vi "SetUpPlotLegend_V0.vi"(1 "Comment":string[](array[string]), 2 "Index":i32[](array[numeric]), 3 "Graph":refnum<vi>) -> ()   [LabVIEW 2021]
panel:
  in  "Graph 2":refnum<vi>
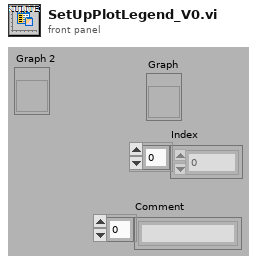
[diagram p1: front panel]
types:
  T1 = cluster{"Start":dbl, "Delta x":dbl, "Data Array out":sgl[][]}
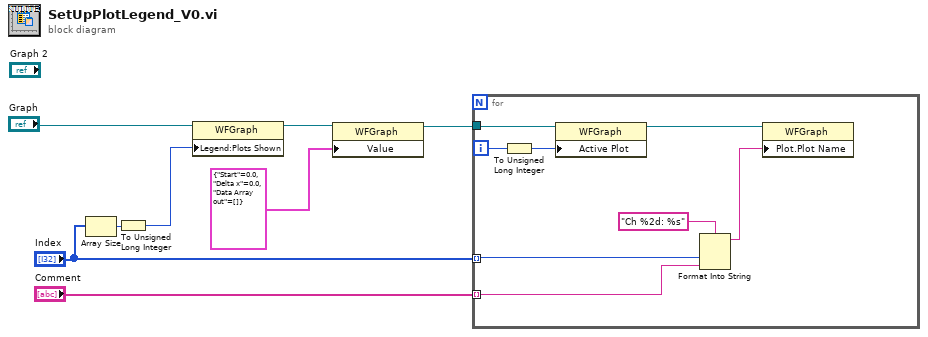
[diagram p0: block diagram]
diagram:
  n1 = Array Size(array="Index") -> (size(s)=w6:i32)
  n2 = To Unsigned Long Integer(number=w6) -> (unsigned 32bit integer=w5:u32)
  n3 = property class="WFGraph"(reference="Graph", "Legend:Plots Shown"=w5) -> (reference out=w3:refnum<vi>)  [unwired: 1 in, 1 out]
  n4 = property class="WFGraph"(reference=w3, "Value"=T1 {"Start"=0.0, "Delta x"=0.0, "Data Array out"=[]}) -> (reference out=w2:refnum<vi>)  [unwired: 1 in, 1 out]
  n5 = for {
    tunnel: w2 -> [w15]
    tunnel: "Index" -> [w12] mode=indexing
    tunnel: "Comment" -> [w11] mode=indexing
    i -> [w16]
    n6 = To Unsigned Long Integer(number=w16) -> (unsigned 32bit integer=w9:u32)
    n7 = property class="WFGraph"(reference=w15, "Active Plot"=w9) -> (reference out=w13:refnum<vi>)  [unwired: 1 in, 1 out]
    n8 = Format Into String(format string="Ch %2d: %s", w12, w11) -> (resulting string=w10:string)  [unwired: 2 in, 1 out]
    n9 = property class="WFGraph"(reference=w13, "Plot.Plot Name"=w10) -> ()  [unwired: 1 in, 2 out]
  }
